vi "Create Tag.vi"(7 "OwnerTree (if Parent empty)":refnum<vi>, 8 "error in (no error)":errorcluster, 9 "Data":variant, 10 "Parent Tag":refnum<class "Tree Tag Class.lvclass">, 11 "Text":string) -> (0 "error out":errorcluster, 2 "Created Tags":refnum<class "Tree Tag Class.lvclass">[](array[class]), 3 "Tag_LVOOP out":refnum<class "Tree Tag Class.lvclass">)   [LabVIEW 2012, in "Tree Tools.lvlib" / "Tree Tag Class.lvclass"]
uses:
  Tree Tag Class.lvclass
  Tree Tag Class.lvclass/Tree Tag Class.ctl
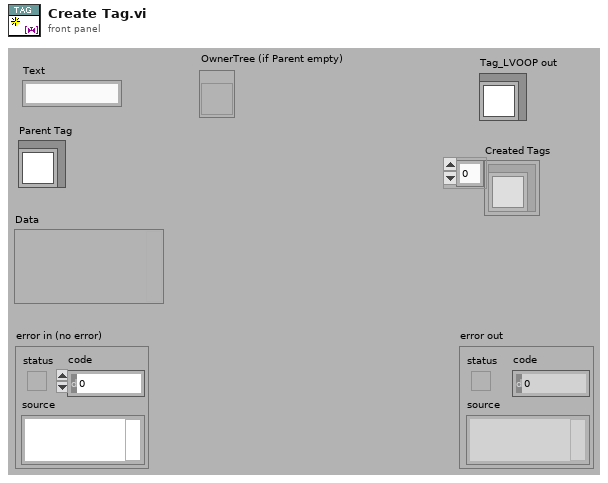
[diagram p1: front panel]
types:
  T1 = cluster{"Parent Tag":refnum<class "Tree Tag Class.lvclass">, "Text":string, "Data":variant}
  T2 = cluster{"Tag_LVOOP in":refnum<class "Tree Tag Class.lvclass">, string, "Variant":variant}
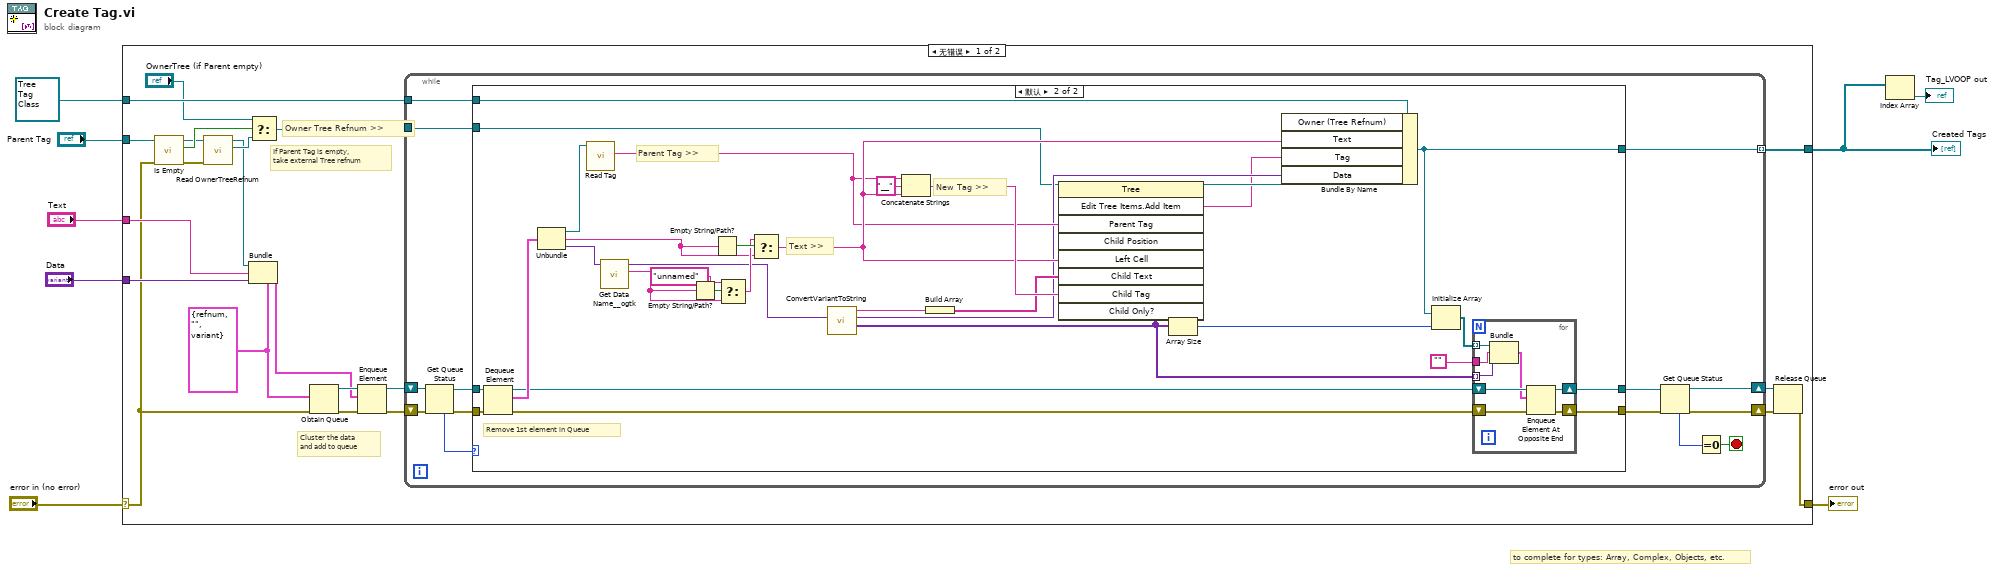
[diagram p0: block diagram]
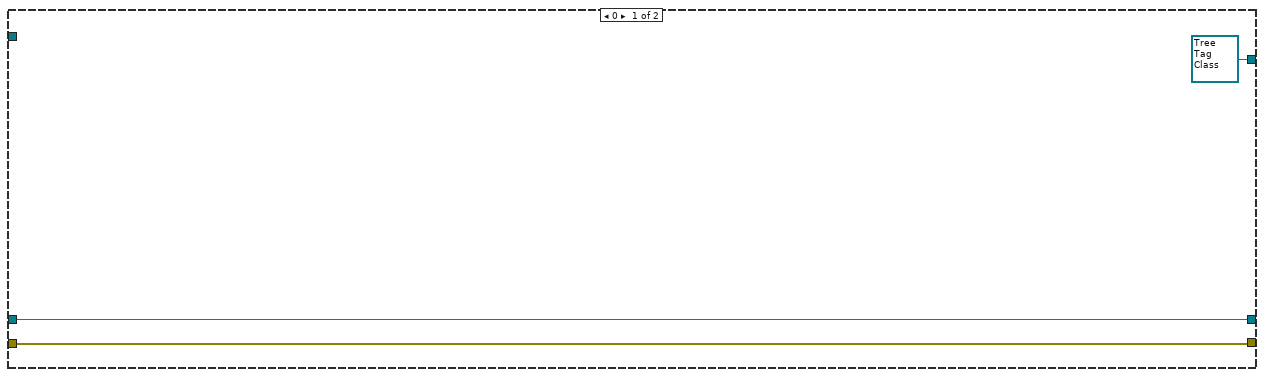
[diagram p2: hidden frame]
diagram:
  # "to complete for types: Array, Complex, Objects, etc."
  n1 = case shown="无错误" "error in (no error)" {
    selector: "error in (no error)" -> [w9 w88]
    tunnel: [w10 w88] -> w7
    tunnel: refnum<class "Tree Tag Class.lvclass"> refnum ("Tag_LVOOP in") -> [w30 _]
    tunnel: "Parent Tag" -> [w29 _]
    tunnel: "Text" -> [w21 _]
    tunnel: "Data" -> [w20 _]
    tunnel: [w19 _] -> w2
    frame No Error {
      w18 = T1 {"Parent Tag"=refnum, "Text"="", "Data"=variant} ("cluster")
      # "Cluster the data\nand add to queue"
      # "If Parent Tag is empty,\ntake external Tree refnum"
      # "Owner Tree Refnum >>"
      n2 = call-dynamic "Is Empty.vi"("error in (no error)"=w9, "Tag_LVOOP in"=w29) -> ("error out"=w22:errorcluster, "Empty"=w26:bool, "Tag_LVOOP out"=w23:refnum<class "Tree Tag Class.lvclass">)  [unwired: 7 out]
      n3 = call-dynamic "Read OwnerTreeRefnum.vi"("error in (no error)"=w22, "Tag_LVOOP.lvclass in"=w23) -> ("Owner (Tree Refnum)"=w27:refnum<vi>, "Tag_LVOOP.lvclass out"=w24:refnum<class "Tree Tag Class.lvclass">)  [unwired: 8 out]
      n4 = Bundle(cluster=w18, "Parent Tag"=w24, "Text"=w21, "Data"=w20) -> (w16:T1)
      n5 = Select(t="OwnerTree (if Parent empty)", s=w26, f=w27) -> (s? t:f=w25:refnum<vi>)
      n6 = Obtain Queue(element data type=w18, error in (no error)=w9) -> (queue out=w17:refnum<queue>, error out=w14:errorcluster)  [unwired: 2 in, 2 out]
      n7 = Enqueue Element(queue=w17, element=w16, error in (no error)=w14) -> (queue out=w15:refnum<queue>, error out=w11:errorcluster)  [unwired: 2 out]
      n8 = while {
        tunnel: w30 -> [w44]
        tunnel: w25 -> [w43]
        tunnel: [w42] -> w19 mode=indexing
        shift-right: [w36] -> w13
        shift-left: w15 -> [w41]
        shift-right: [w32] -> w12
        shift-left: w11 -> [w31]
        stop <- w35 stop-if-true
        n9 = Get Queue Status(queue=w41, error in (no error)=w31) -> (queue out=w39:refnum<queue>, error out=w40:errorcluster, # elements in queue=w38:i32)  [unwired: 6 out]
        n10 = case shown="默认" w38 {
          tunnel: w44 -> [_ w79]
          tunnel: w43 -> [_ w50]
          tunnel: [refnum<class "Tree Tag Class.lvclass"> refnum ("Tag_LVOOP in") w65] -> w42
          tunnel: w40 -> [w45 w57]
          tunnel: w39 -> [w47 w56]
          tunnel: [w47 w53] -> w37
          tunnel: [w45 w52] -> w33
          frame 0 {
          }
          frame Default {
            # "Remove 1st element in Queue"
            # "Text >>"
            # "Parent Tag >>"
            # "New Tag >>"
            n11 = Dequeue Element(queue=w56, error in (no error)=w57) -> (queue out=w54:refnum<queue>, element=w55:T1, error out=w51:errorcluster)  [unwired: 2 out]
            n12 = Unbundle(w55) -> ("Parent Tag"=w76:refnum<class "Tree Tag Class.lvclass">, "Text"=w70:string, "Data"=w71:variant)
            n13 = call-dynamic "Read Tag.vi"("Tag_LVOOP.lvclass in"=w76) -> ("Tag"=w67:string)  [unwired: 1 in, 9 out]
            n14 = call <userlib>:"Get Data Name__ogtk.vi"("Data"=w71) -> ("Data Name"=w69:string, "Data dup"=w60:variant)  [unwired: 8 in, 1 out]
            n15 = Empty String/Path?(string/path=w69) -> (empty?=w74:bool)
            n16 = Empty String/Path?(string/path=w70) -> (empty?=w75:bool)
            n17 = Select(t="unnamed", s=w74, f=w69) -> (s? t:f=w73:string)
            n18 = Select(t=w73, s=w75, f=w70) -> (s? t:f=w68:string)
            n19 = call "ConvertVariantToString.vi"("Variant"=w60) -> ("Array of VData"=w58:variant[], "Variant dup"=w59:variant, "String"=w61:string)  [unwired: 3 in, 5 out]
            n20 = Concatenate Strings(w67, "__" ("string"), w68) -> (w77:string)
            n21 = Build Array(w61) -> (w62:string[])
            n22 = invoke class="Tree" method="Edit Tree Items.Add Item"(reference=w50, "Parent Tag"=w67, "Left Cell"=w68, "Child Text"=w62, "Child Tag"=w77) -> (reference out=w49:refnum<vi>, "Edit Tree Items:Add Item"=w48:string)  [unwired: 4 in, 7 out]
            n23 = Array Size(array=w58) -> (size(s)=w66:i32)
            n24 = Bundle By Name(cluster=w79, "Owner (Tree Refnum)"=w49, "Text"=w68, "Tag"=w48, "Data"=w59) -> (w65:refnum<class "Tree Tag Class.lvclass">)
            n25 = Initialize Array(w65, w66) -> (w64:refnum<class "Tree Tag Class.lvclass">[])
            n26 = for {
              tunnel: w64 -> [w87] mode=indexing
              tunnel: "" -> [w86]
              tunnel: w58 -> [w85] mode=indexing
              shift-right: [w82] -> w53
              shift-left: w54 -> [w84]
              shift-right: [w81] -> w52
              shift-left: w51 -> [w80]
              n27 = Bundle("Tag_LVOOP in"=w87, w86, "Variant"=w85) -> (w83:T2)  [unwired: 1 out]
              n28 = Enqueue Element At Opposite End(queue=w84, element=w83, error in (no error)=w80) -> (queue out=w82:refnum<queue>, error out=w81:errorcluster)  [unwired: 2 out]
            }
          }
        }
        n29 = Get Queue Status(queue=w37, error in (no error)=w33) -> (queue out=w36:refnum<queue>, error out=w32:errorcluster, # elements in queue=w34:i32)  [unwired: 6 out]
        n30 = Equal To 0?(x=w34) -> (x = 0?=w35:bool)
      }
      n31 = Release Queue(queue=w13, error in (no error)=w12) -> (error out=w10:errorcluster)  [unwired: 3 out]
    }
    frame Error {
    }
  }
  "error out" <- w7
  "Created Tags" <- w2
  n32 = Index Array(array=w2) -> (element=→"Tag_LVOOP out":refnum<class "Tree Tag Class.lvclass">)  [unwired: 1 in]
